vi "标定数据保存.vi"(11 "枚举":enum16{"Read", "Write"}(ring)) -> ()   [LabVIEW 2019]
uses:
  Global_Variable/Global.vi
panel:
  out "工位二扭矩偏移":cluster{"正向":dbl, "逆向":dbl}
  out "工位一扭矩偏移":cluster{"正向":dbl, "逆向":dbl}
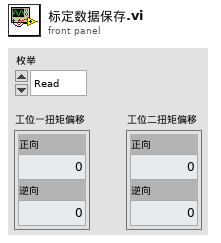
[diagram p1: front panel]
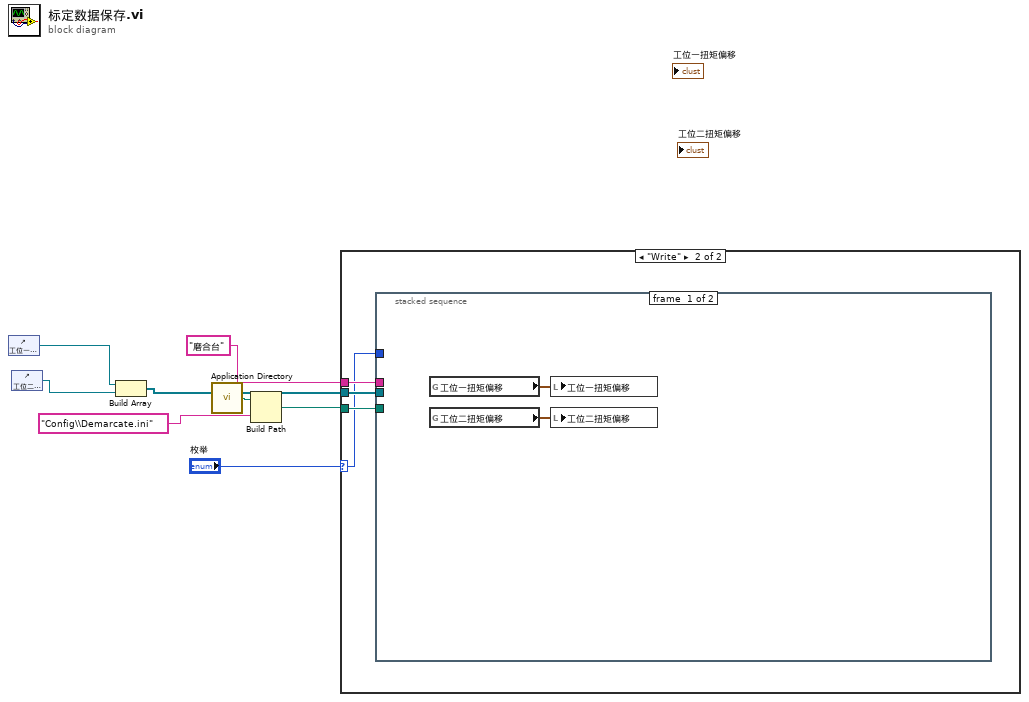
[diagram p0: block diagram]
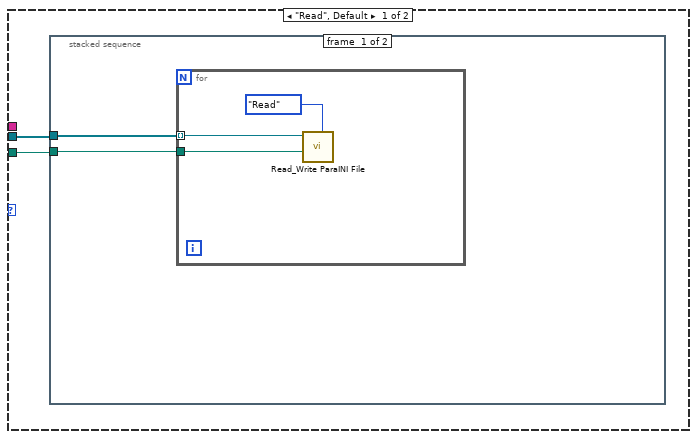
[diagram p2: hidden frame]
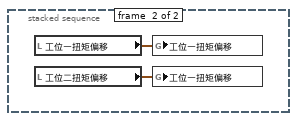
[diagram p3: hidden frame]
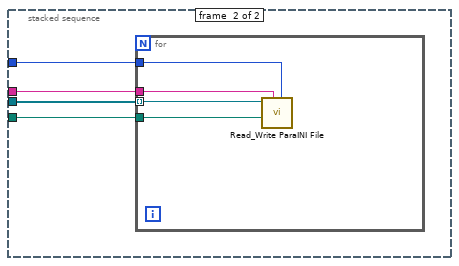
[diagram p4: hidden frame]
diagram:
  n1 = control-ref of="工位一扭矩偏移"() -> (w6:refnum<vi>)
  n2 = control-ref of="工位二扭矩偏移"() -> (w7:refnum<vi>)
  n3 = Build Array(w6, w7) -> (w5:refnum<vi>[])
  n4 = call <vilib>:"Application Directory.vi"() -> ("Application Directory"=w4:path)
  n5 = Build Path(base path=w4, name or relative path="Config\\Demarcate.ini" ("名称或相对路径")) -> (appended path=w2:path)
  n6 = case shown="\"Write\"" "枚举" {
    selector: "枚举" -> [_ w18]
    tunnel: w5 -> [w10 w21]
    tunnel: w2 -> [w9 w20]
    tunnel: "磨合台" -> [_ w19]
    frame "Read", Default {
      n7 = stacked-sequence {
        tunnel: w10 -> [w12 _]
        tunnel: w9 -> [w11 _]
        frame #0 {
          n8 = for {
            tunnel: w12 -> [w15] mode=indexing
            tunnel: w11 -> [w14]
            n9 = call "Read_Write ParaINI File.vi"("Mode"=enum16{"Read", "Write"}."Read", "Filepath"=w14, "Ctl Refnum"=w15) -> ()  [unwired: 8 in, 1 out]
          }
        }
        frame #1 {
          n10 = local read "工位一扭矩偏移"() -> (w17:cluster{"正向":dbl, "逆向":dbl})
          n11 = local read "工位二扭矩偏移"() -> (w16:cluster{"正向":dbl, "逆向":dbl})
          n12 = global write "Global.vi" "工位一扭矩偏移"(w17) -> ()
          n13 = global write "Global.vi" "工位一扭矩偏移"(w16) -> ()
        }
      }
    }
    frame "Write" {
      n14 = stacked-sequence {
        tunnel: w21 -> [_ w27]
        tunnel: w20 -> [_ w26]
        tunnel: w19 -> [_ w25]
        tunnel: w18 -> [_ w24]
        frame #0 {
          n15 = global read "Global.vi" "工位一扭矩偏移"() -> (w23:cluster{"正向":dbl, "逆向":dbl})
          n16 = global read "Global.vi" "工位二扭矩偏移"() -> (w22:cluster{"正向":dbl, "逆向":dbl})
          n17 = local write "工位一扭矩偏移"(w23) -> ()
          n18 = local write "工位二扭矩偏移"(w22) -> ()
        }
        frame #1 {
          n19 = for {
            tunnel: w27 -> [w29] mode=indexing
            tunnel: w26 -> [w28]
            tunnel: w25 -> [w30]
            tunnel: w24 -> [w31]
            n20 = call "Read_Write ParaINI File.vi"("Mode"=w31, "Section"=w30, "Filepath"=w28, "Ctl Refnum"=w29) -> ()  [unwired: 7 in, 1 out]
          }
        }
      }
    }
  }
